vi "Voice coil and camera trigger.vi"() -> ()   [LabVIEW 2020]
uses:
  <vilib>/DAQmx/write.llb/DAQmx Write (Analog 1D Wfm NChan NSamp).vi
  <vilib>/DAQmx/create/channels.llb/DAQmx Create Channel (AO-Voltage-Basic).vi
  <vilib>/DAQmx/configure/timing.llb/DAQmx Timing (Use Waveform).vi
  <vilib>/DAQmx/miscellaneous.llb/DAQmx Fill In Error Info.vi
  <vilib>/measure/NI_MABase.lvlib
panel:
  in  "Stop 2":bool
  out "LabVIEW generated Sawtooth input (blue) and Camera trigger (red)":waveform(dbl)[](graph)=[{"t0"=timestamp(0 s since 1904-01-01), "dt"=0.001, "Y"=array[1000 elements]}, {"t0"=timestamp(0 s since 1904-01-01), "dt"=0.001, "Y"=array[1000 elements]}]
  in  "Sawtooth Offset (mv)":dbl format="%.2p"
  in  "Camera trigger delay (degrees)":dbl format="%.2p"
  in  "Exposure time (ms)":dbl=1000.0
  out "# Samples written per channel":u32=1000
  in  "Sawtooth Phase":dbl=180.0 format="%.2p"
  in  "Sawtooth Amplitude (mv)":dbl format="%.2p"
  # "Sawtooth signal has to be smooth around the edges"
  # "Fs= sampling rate in samples per second\n#s= number of samples in the waveform"
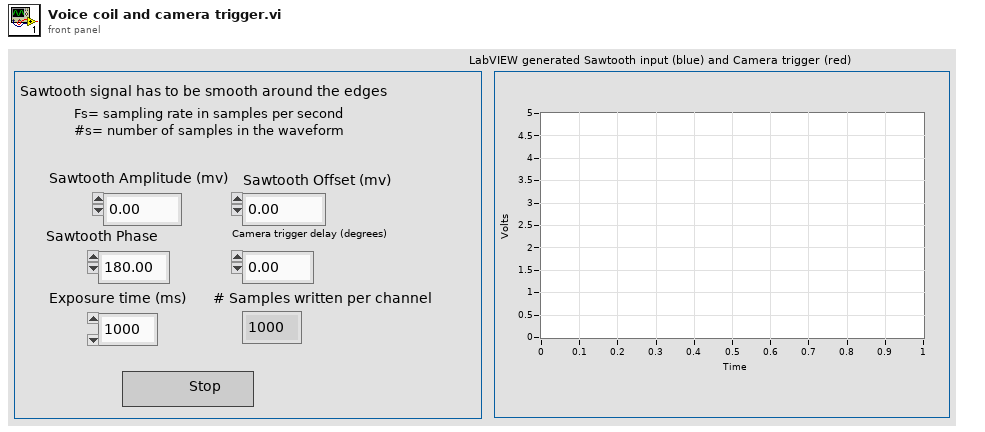
[diagram p1: front panel]
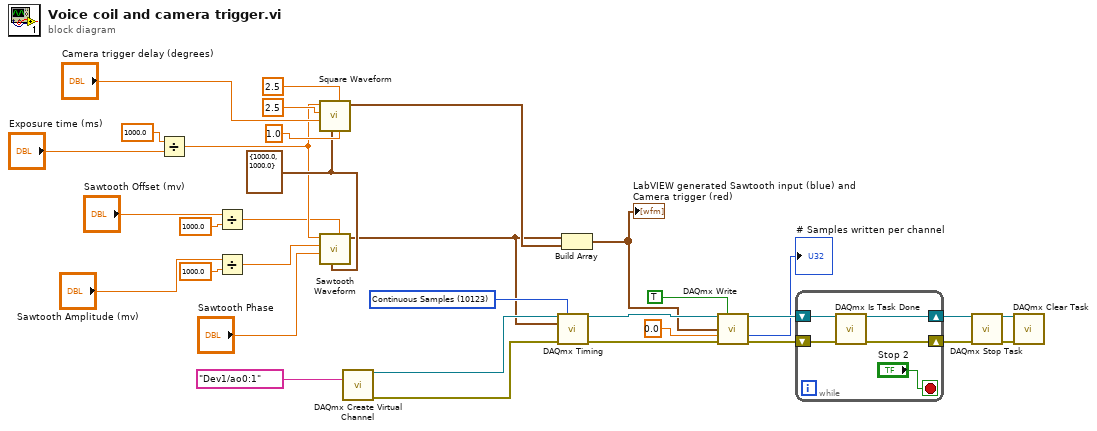
[diagram p0: block diagram]
diagram:
  w12 = cluster{"Fs":dbl, "#s":dbl} {"Fs"=1000.0, "#s"=1000.0} ("sampling info")
  w28 = 10123 items=["Finite Samples"=10178, "Continuous Samples"=10123, "Hardware Timed Single Point"=12522] ("sample mode")
  n1 = Divide(x=1000.0, y="Exposure time (ms)") -> (x/y=w9:dbl)
  n2 = Divide(x="Sawtooth Offset (mv)", y=1000.0) -> (x/y=w6:dbl)
  n3 = Divide(x="Sawtooth Amplitude (mv)", y=1000.0) -> (x/y=w1:dbl)
  n4 = call <vilib>:"Square Waveform.vi"("duty cycle (%)"=1.0, "offset"=2.5, "sampling info"=w12, "phase"="Camera trigger delay (degrees)", "amplitude"=2.5, "frequency"=w9) -> ("signal out"=w13:waveform(dbl))  [unwired: 4 in, 1 out]
  n5 = call <vilib>:"Sawtooth Waveform.vi"("offset"=w6, "sampling info"=w12, "phase"="Sawtooth Phase", "amplitude"=w1, "frequency"=w9) -> ("signal out"=w7:waveform(dbl))  [unwired: 5 in, 1 out]
  n6 = call-poly <vilib>:"DAQmx Create Virtual Channel.vi"("physical channels"=tag "Dev1/ao0:1") -> ("task out"=w30:refnum<k21>, "error out"=w29:errorcluster)  [unwired: 13 in]
  n7 = call-poly <vilib>:"DAQmx Timing.vi"("task/channels in"=w30, "sample mode"=w28, "waveform"=w7, "error in"=w29) -> ("task out"=w25:refnum<k21>, "error out"=w24:errorcluster)  [unwired: 10 in]
  n8 = Build Array(w7, w13) -> (w8:waveform(dbl)[])
  "LabVIEW generated Sawtooth input (blue) and Camera trigger (red)" <- w8
  n9 = call-poly <vilib>:"DAQmx Write.vi"("task/channels in"=w25, "auto start"=TRUE, "data"=w8, "timeout"=0.0, "error in"=w24) -> ("task out"=w26:refnum<k21>, "number of samples written per channel"=→"# Samples written per channel":u32, "error out"=w27:errorcluster)  [unwired: 8 in]
  n10 = while {
    shift-right: [w35] -> w21
    shift-left: w26 -> [w38]
    shift-right: [w36] -> w22
    shift-left: w27 -> [w37]
    stop <- "Stop 2" stop-if-true
    n11 = call <vilib>:"DAQmx Is Task Done.vi"("task/channels in"=w38, "error in"=w37) -> ("task out"=w35:refnum<k21>, "error out"=w36:errorcluster)  [unwired: 11 in, 1 out]
  }
  n12 = call <vilib>:"DAQmx Stop Task.vi"("task/channels in"=w21, "error in"=w22) -> ("task out"=w31:refnum<k21>, "error out"=w32:errorcluster)  [unwired: 12 in]
  n13 = call <vilib>:"DAQmx Clear Task.vi"("task in"=w31, "error in"=w32) -> ()  [unwired: 13 in, 1 out]
